vi "Predict(Dataset).vi"(6 "Dataset":T29={"Dataset_Size"=0, "Dims_In"={"C"=0, "H"=0, "W"=0}, "Labels"=[], "File Paths"=[], "Outputs Ref."=refnum, "Inputs Ref."=variant(refnum<data-value> refnum), "Dims_Out"={"C"=0, "H"=0, "W"=0}}, 8 "error in (no error)":errorcluster, 10 "Feature Scorer Params":T27, 11 "PCore_Instance in":T1={"Dataset_Stats"={"means"={"R"=0.0, "G"=0.0, "B"=0.0}, "vars"={"R"=0.0, "G"=0.0, "B"=0.0}, "DS_Size"=0}, "NN"={"Name"="", "No of Layers"=0, "mBatch"=0, "Layers"=[], "Dimty"=enum."In1D_Out1D", "Dims_In"={"C"=0, "H"=0, "W"=0}, "Dims_Out"={"C"=0, "H"=0, "W"=0}, "Working_Dir"=path "", "Train?"=FALSE, "Train_Params"={"Optimizer"=enum."SGD", "Beta_1"=0.0, "Beta_2"=0.0, "Weight Decay(L1)"=0.0, "Weight Decay(L2)"=0.0, "Data_Sampling"=enum."Random"}, "LR_Update_Policy"={"Policy_Type"=enum."Manual", "LR0"=0.0, "k"=0.0, "WarmUp_Policy"=enum."Step", "WarmUp_Iter"=0, "WarmUp_Ratio"=0.0}, "Session Data"={"Epochs"=0.0, "Tot_Iter"=0, "LR"=0.0, "LR_iter"=0}, "Ground_truth"={"Y"=variant}, "NNg_hdls"={"cudnn"=0, "cublas"=0, "stream"=0, "curand"=0}, "NN_Device"=enum."CPU", "GPU Id"=0, "Labels"=[], "Receptive Field"=[], "Loss_Type"=enum."None", "Loss_Cfg_Prms"=variant, "NNG_WS"={"NNG_WS_Mem"=refnum, "Max_WS_Size"=0}}, "PCore_Device"=enum."CPU", "PatchCore_Init_CFG"={"BackBone"=enum."WRN_50_2_L2L3", "Out_Layers_Names"=[], "Patch_Size"=0}, "Coreset Params"={"Sampling_Ratio"=0.0, "Startd_idx"=0, "Random_Proj?"=FALSE, "Rnd. Proj. Params"={"Proj._Dim."=0, "Epsilon"=0.9, "Seed"=42}}, "MemBank_Data"={"MemBank"=variant, "MemBank Norm"=variant}} {"NN out"."LR_Update_Policy"."WarmUp_Ratio" min=1; "NN out"."LR_Update_Policy"."WarmUp_Iter" min=1; "NN out"."LR_Update_Policy"."LR0" format="%.7f"; "Dataset_Stats"."vars"."R" format="%#_3g"; "Dataset_Stats"."vars"."G" format="%#_3g"; "Dataset_Stats"."vars"."B" format="%#_3g"; "Dataset_Stats"."means"."R" format="%#_3g"; "Dataset_Stats"."means"."G" format="%#_3g"; "Dataset_Stats"."means"."B" format="%#_3g"}) -> (0 "error out":errorcluster, 1 "anomaly maps":sgl[][][](array[numeric]), 2 "pred scores":sgl[](array[numeric]), 3 "PCore_Instance out":T1={"Dataset_Stats"={"means"={"R"=0.66, "G"=0.59, "B"=0.44}, "vars"={"R"=0.66, "G"=0.59, "B"=0.44}, "DS_Size"=0}, "NN"={"Name"="wrn", "No of Layers"=63, "mBatch"=1, "Layers"=[refnum, refnum, refnum, refnum, refnum, refnum, refnum, refnum, refnum, refnum, refnum, refnum, refnum, refnum, refnum, refnum, refnum, refnum, refnum, refnum, refnum, refnum, refnum, refnum, refnum, refnum, refnum, refnum, refnum, refnum, refnum, refnum, refnum, refnum, refnum, refnum, refnum, refnum, refnum, refnum, refnum, refnum, refnum, refnum, refnum, refnum, refnum, refnum, refnum, refnum, refnum, refnum, refnum, refnum, refnum, refnum, refnum, refnum, refnum, refnum, refnum, refnum, refnum], "Dimty"=enum."In3D_Out3D", "Dims_In"={"C"=3, "H"=224, "W"=224}, "Dims_Out"={"C"=302, "H"=28, "W"=28}, "Working_Dir"=path "D:/Ngene/Projects_SVN/DeepLTK/R_and_D/2024_02_01_Patchcore/LabVIEW/PatchCore_v5.0/working/wrn", "Train?"=FALSE, "Train_Params"={"Optimizer"=enum."SGD", "Beta_1"=0.999, "Beta_2"=0.999, "Weight Decay(L1)"=0.0, "Weight Decay(L2)"=0.0, "Data_Sampling"=enum."Random"}, "LR_Update_Policy"={"Policy_Type"=enum."Manual", "LR0"=0.0, "k"=0.0, "WarmUp_Policy"=enum."Step", "WarmUp_Iter"=100, "WarmUp_Ratio"=10.0}, "Session Data"={"Epochs"=0.0, "Tot_Iter"=1, "LR"=0.0, "LR_iter"=1}, "Ground_truth"={"Y"=variant(refnum<data-value> refnum)}, "NNg_hdls"={"cudnn"=2143106709504, "cublas"=2177817002560, "stream"=2141212075440, "curand"=2143055681792}, "NN_Device"=enum."GPU", "GPU Id"=0, "Labels"=["tench", "goldfish", "great white shark", "tiger shark", "hammerhead", "electric ray", "stingray", "cock", "hen", "ostrich", "brambling", "goldfinch", "house finch", "junco", "indigo bunting", "robin", "bulbul", "jay", "magpie", "chickadee", "water ouzel", "kite", "bald eagle", "vulture", "great grey owl", "European fire salamander", "common newt", "eft", "spotted salamander", "axolotl", "bullfrog", "tree frog", "tailed frog", "loggerhead", "leatherback turtle", "mud turtle", "terrapin", "box turtle", "banded gecko", "common iguana", "American chameleon", "whiptail", "agama", "frilled lizard", "alligator lizard", "Gila monster", "green lizard", "African chameleon", "Komodo dragon", "African crocodile", "American alligator", "triceratops", "thunder snake", "ringneck snake", "hognose snake", "green snake", "king snake", "garter snake", "water snake", "vine snake", "night snake", "boa constrictor", "rock python", "Indian cobra", "green mamba", "sea snake", "horned viper", "diamondback", "sidewinder", "trilobite", "harvestman", "scorpion", "black and gold garden spider", "barn spider", "garden spider", "black widow", "tarantula", "wolf spider", "tick", "centipede", "black grouse", "ptarmigan", "ruffed grouse", "prairie chicken", "peacock", "quail", "partridge", "African grey", "macaw", "sulphur-crested cockatoo", "lorikeet", "coucal", "bee eater", "hornbill", "hummingbird", "jacamar", "toucan", "drake", "red-breasted merganser", "goose", "black swan", "tusker", "echidna", "platypus", "wallaby", "koala", "wombat", "jellyfish", "sea anemone", "brain coral", "flatworm", "nematode", "conch", "snail", "slug", "sea slug", "chiton", "chambered nautilus", "Dungeness crab", "rock crab", "fiddler crab", "king crab", "American lobster", "spiny lobster", "crayfish", "hermit crab", "isopod", "white stork", "black stork", "spoonbill", "flamingo", "little blue heron", "American egret", "bittern", "crane", "limpkin", "European gallinule", "American coot", "bustard", "ruddy turnstone", "red-backed sandpiper", "redshank", "dowitcher", "oystercatcher", "pelican", "king penguin", "albatross", "grey whale", "killer whale", "dugong", "sea lion", "Chihuahua", "Japanese spaniel", "Maltese dog", "Pekinese", "Shih-Tzu", "Blenheim spaniel", "papillon", "toy terrier", "Rhodesian ridgeback", "Afghan hound", "basset", "beagle", "bloodhound", "bluetick", "black-and-tan coonhound", "Walker hound", "English foxhound", "redbone", "borzoi", "Irish wolfhound", "Italian greyhound", "whippet", "Ibizan hound", "Norwegian elkhound", "otterhound", "Saluki", "Scottish deerhound", "Weimaraner", "Staffordshire bullterrier", "American Staffordshire terrier", "Bedlington terrier", "Border terrier", "Kerry blue terrier", "Irish terrier", "Norfolk terrier", "Norwich terrier", "Yorkshire terrier", "wire-haired fox terrier", "Lakeland terrier", "Sealyham terrier", "Airedale", "cairn", "Australian terrier", "Dandie Dinmont", "Boston bull", "miniature schnauzer", "giant schnauzer", "standard schnauzer", "Scotch terrier", "Tibetan terrier", "silky terrier", "soft-coated wheaten terrier", "West Highland white terrier", "Lhasa", "flat-coated retriever", "curly-coated retriever", "golden retriever", "Labrador retriever", "Chesapeake Bay retriever", "German short-haired pointer", "vizsla", "English setter", "Irish setter", "Gordon setter", "Brittany spaniel", "clumber", "English springer", "Welsh springer spaniel", "cocker spaniel", "Sussex spaniel", "Irish water spaniel", "kuvasz", "schipperke", "groenendael", "malinois", "briard", "kelpie", "komondor", "Old English sheepdog", "Shetland sheepdog", "collie", "Border collie", "Bouvier des Flandres", "Rottweiler", "German shepherd", "Doberman", "miniature pinscher", "Greater Swiss Mountain dog", "Bernese mountain dog", "Appenzeller", "EntleBucher", "boxer", "bull mastiff", "Tibetan mastiff", "French bulldog", "Great Dane", "Saint Bernard", "Eskimo dog", "malamute", "Siberian husky", "dalmatian", "affenpinscher", "basenji", "pug", "Leonberg", "Newfoundland", "Great Pyrenees", "Samoyed", "Pomeranian", "chow", "keeshond", "Brabancon griffon", "Pembroke", "Cardigan", "toy poodle", "miniature poodle", "standard poodle", "Mexican hairless", "timber wolf", "white wolf", "red wolf", "coyote", "dingo", "dhole", "African hunting dog", "hyena", "red fox", "kit fox", "Arctic fox", "grey fox", "tabby", "tiger cat", "Persian cat", "Siamese cat", "Egyptian cat", "cougar", "lynx", "leopard", "snow leopard", "jaguar", "lion", "tiger", "cheetah", "brown bear", "American black bear", "ice bear", "sloth bear", "mongoose", "meerkat", "tiger beetle", "ladybug", "ground beetle", "long-horned beetle", "leaf beetle", "dung beetle", "rhinoceros beetle", "weevil", "fly", "bee", "ant", "grasshopper", "cricket", "walking stick", "cockroach", "mantis", "cicada", "leafhopper", "lacewing", "dragonfly", "damselfly", "admiral", "ringlet", "monarch", "cabbage butterfly", "sulphur butterfly", "lycaenid", "starfish", "sea urchin", "sea cucumber", "wood rabbit", "hare", "Angora", "hamster", "porcupine", "fox squirrel", "marmot", "beaver", "guinea pig", "sorrel", "zebra", "hog", "wild boar", "warthog", "hippopotamus", "ox", "water buffalo", "bison", "ram", "bighorn", "ibex", "hartebeest", "impala", "gazelle", "Arabian camel", "llama", "weasel", "mink", "polecat", "black-footed ferret", "otter", "skunk", "badger", "armadillo", "three-toed sloth", "orangutan", "gorilla", "chimpanzee", "gibbon", "siamang", "guenon", "patas", "baboon", "macaque", "langur", "colobus", "proboscis monkey", "marmoset", "capuchin", "howler monkey", "titi", "spider monkey", "squirrel monkey", "Madagascar cat", "indri", "Indian elephant", "African elephant", "lesser panda", "giant panda", "barracouta", "eel", "coho", "rock beauty", "anemone fish", "sturgeon", "gar", "lionfish", "puffer", "abacus", "abaya", "academic gown", "accordion", "acoustic guitar", "aircraft carrier", "airliner", "airship", "altar", "ambulance", "amphibian", "analog clock", "apiary", "apron", "ashcan", "assault rifle", "backpack", "bakery", "balance beam", "balloon", "ballpoint", "Band Aid", "banjo", "bannister", "barbell", "barber chair", "barbershop", "barn", "barometer", "barrel", "barrow", "baseball", "basketball", "bassinet", "bassoon", "bathing cap", "bath towel", "bathtub", "beach wagon", "beacon", "beaker", "bearskin", "beer bottle", "beer glass", "bell cote", "bib", "bicycle-built-for-two", "bikini", "binder", "binoculars", "birdhouse", "boathouse", "bobsled", "bolo tie", "bonnet", "bookcase", "bookshop", "bottlecap", "bow", "bow tie", "brass", "brassiere", "breakwater", "breastplate", "broom", "bucket", "buckle", "bulletproof vest", "bullet train", "butcher shop", "cab", "caldron", "candle", "cannon", "canoe", "can opener", "cardigan", "car mirror", "carousel", "carpenter's kit", "carton", "car wheel", "cash machine", "cassette", "cassette player", "castle", "catamaran", "CD player", "cello", "cellular telephone", "chain", "chainlink fence", "chain mail", "chain saw", "chest", "chiffonier", "chime", "china cabinet", "Christmas stocking", "church", "cinema", "cleaver", "cliff dwelling", "cloak", "clog", "cocktail shaker", "coffee mug", "coffeepot", "coil", "combination lock", "computer keyboard", "confectionery", "container ship", "convertible", "corkscrew", "cornet", "cowboy boot", "cowboy hat", "cradle", "crane", "crash helmet", "crate", "crib", "Crock Pot", "croquet ball", "crutch", "cuirass", "dam", "desk", "desktop computer", "dial telephone", "diaper", "digital clock", "digital watch", "dining table", "dishrag", "dishwasher", "disk brake", "dock", "dogsled", "dome", "doormat", "drilling platform", "drum", "drumstick", "dumbbell", "Dutch oven", "electric fan", "electric guitar", "electric locomotive", "entertainment center", "envelope", "espresso maker", "face powder", "feather boa", "file", "fireboat", "fire engine", "fire screen", "flagpole", "flute", "folding chair", "football helmet", "forklift", "fountain", "fountain pen", "four-poster", "freight car", "French horn", "frying pan", "fur coat", "garbage truck", "gasmask", "gas pump", "goblet", "go-kart", "golf ball", "golfcart", "gondola", "gong", "gown", "grand piano", "greenhouse", "grille", "grocery store", "guillotine", "hair slide", "hair spray", "half track", "hammer", "hamper", "hand blower", "hand-held computer", "handkerchief", "hard disc", "harmonica", "harp", "harvester", "hatchet", "holster", "home theater", "honeycomb", "hook", "hoopskirt", "horizontal bar", "horse cart", "hourglass", "iPod", "iron", "jack-o'-lantern", "jean", "jeep", "jersey", "jigsaw puzzle", "jinrikisha", "joystick", "kimono", "knee pad", "knot", "lab coat", "ladle", "lampshade", "laptop", "lawn mower", "lens cap", "letter opener", "library", "lifeboat", "lighter", "limousine", "liner", "lipstick", "Loafer", "lotion", "loudspeaker", "loupe", "lumbermill", "magnetic compass", "mailbag", "mailbox", "maillot", "maillot", "manhole cover", "maraca", "marimba", "mask", "matchstick", "maypole", "maze", "measuring cup", "medicine chest", "megalith", "microphone", "microwave", "military uniform", "milk can", "minibus", "miniskirt", "minivan", "missile", "mitten", "mixing bowl", "mobile home", "Model T", "modem", "monastery", "monitor", "moped", "mortar", "mortarboard", "mosque", "mosquito net", "motor scooter", "mountain bike", "mountain tent", "mouse", "mousetrap", "moving van", "muzzle", "nail", "neck brace", "necklace", "nipple", "notebook", "obelisk", "oboe", "ocarina", "odometer", "oil filter", "organ", "oscilloscope", "overskirt", "oxcart", "oxygen mask", "packet", "paddle", "paddlewheel", "padlock", "paintbrush", "pajama", "palace", "panpipe", "paper towel", "parachute", "parallel bars", "park bench", "parking meter", "passenger car", "patio", "pay-phone", "pedestal", "pencil box", "pencil sharpener", "perfume", "Petri dish", "photocopier", "pick", "pickelhaube", "picket fence", "pickup", "pier", "piggy bank", "pill bottle", "pillow", "ping-pong ball", "pinwheel", "pirate", "pitcher", "plane", "planetarium", "plastic bag", "plate rack", "plow", "plunger", "Polaroid camera", "pole", "police van", "poncho", "pool table", "pop bottle", "pot", "potter's wheel", "power drill", "prayer rug", "printer", "prison", "projectile", "projector", "puck", "punching bag", "purse", "quill", "quilt", "racer", "racket", "radiator", "radio", "radio telescope", "rain barrel", "recreational vehicle", "reel", "reflex camera", "refrigerator", "remote control", "restaurant", "revolver", "rifle", "rocking chair", "rotisserie", "rubber eraser", "rugby ball", "rule", "running shoe", "safe", "safety pin", "saltshaker", "sandal", "sarong", "sax", "scabbard", "scale", "school bus", "schooner", "scoreboard", "screen", "screw", "screwdriver", "seat belt", "sewing machine", "shield", "shoe shop", "shoji", "shopping basket", "shopping cart", "shovel", "shower cap", "shower curtain", "ski", "ski mask", "sleeping bag", "slide rule", "sliding door", "slot", "snorkel", "snowmobile", "snowplow", "soap dispenser", "soccer ball", "sock", "solar dish", "sombrero", "soup bowl", "space bar", "space heater", "space shuttle", "spatula", "speedboat", "spider web", "spindle", "sports car", "spotlight", "stage", "steam locomotive", "steel arch bridge", "steel drum", "stethoscope", "stole", "stone wall", "stopwatch", "stove", "strainer", "streetcar", "stretcher", "studio couch", "stupa", "submarine", "suit", "sundial", "sunglass", "sunglasses", "sunscreen", "suspension bridge", "swab", "sweatshirt", "swimming trunks", "swing", "switch", "syringe", "table lamp", "tank", "tape player", "teapot", "teddy", "television", "tennis ball", "thatch", "theater curtain", "thimble", "thresher", "throne", "tile roof", "toaster", "tobacco shop", "toilet seat", "torch", "totem pole", "tow truck", "toyshop", "tractor", "trailer truck", "tray", "trench coat", "tricycle", "trimaran", "tripod", "triumphal arch", "trolleybus", "trombone", "tub", "turnstile", "typewriter keyboard", "umbrella", "unicycle", "upright", "vacuum", "vase", "vault", "velvet", "vending machine", "vestment", "viaduct", "violin", "volleyball", "waffle iron", "wall clock", "wallet", "wardrobe", "warplane", "washbasin", "washer", "water bottle", "water jug", "water tower", "whiskey jug", "whistle", "wig", "window screen", "window shade", "Windsor tie", "wine bottle", "wing", "wok", "wooden spoon", "wool", "worm fence", "wreck", "yawl", "yurt", "web site", "comic book", "crossword puzzle", "street sign", "traffic light", "book jacket", "menu", "plate", "guacamole", "consomme", "hot pot", "trifle", "ice cream", "ice lolly", "French loaf", "bagel", "pretzel", "cheeseburger", "hotdog", "mashed potato", "head cabbage", "broccoli", "cauliflower", "zucchini", "spaghetti squash", "acorn squash", "butternut squash", "cucumber", "artichoke", "bell pepper", "cardoon", "mushroom", "Granny Smith", "strawberry", "orange", "lemon", "fig", "pineapple", "banana", "jackfruit", "custard apple", "pomegranate", "hay", "carbonara", "chocolate sauce", "dough", "meat loaf", "pizza", "potpie", "burrito", "red wine", "espresso", "cup", "eggnog", "alp", "bubble", "cliff", "coral reef", "geyser", "lakeside", "promontory", "sandbar", "seashore", "valley", "volcano", "ballplayer", "groom", "scuba diver", "rapeseed", "daisy", "yellow lady's slipper", "corn", "acorn", "hip", "buckeye", "coral fungus", "agaric", "gyromitra", "stinkhorn", "earthstar", "hen-of-the-woods", "bolete", "ear", "toilet tissue"], "Receptive Field"=[{"V"=1, "H"=1}, {"V"=7, "H"=7}, {"V"=9, "H"=9}, {"V"=9, "H"=9}, {"V"=21, "H"=21}, {"V"=21, "H"=21}, {"V"=9, "H"=9}, {"V"=21, "H"=21}, {"V"=21, "H"=21}, {"V"=33, "H"=33}, {"V"=33, "H"=33}, {"V"=33, "H"=33}, {"V"=33, "H"=33}, {"V"=45, "H"=45}, {"V"=45, "H"=45}, {"V"=45, "H"=45}, {"V"=45, "H"=45}, {"V"=57, "H"=57}, {"V"=57, "H"=57}, {"V"=45, "H"=45}, {"V"=57, "H"=57}, {"V"=57, "H"=57}, {"V"=81, "H"=81}, {"V"=81, "H"=81}, {"V"=81, "H"=81}, {"V"=81, "H"=81}, {"V"=105, "H"=105}, {"V"=105, "H"=105}, {"V"=105, "H"=105}, {"V"=105, "H"=105}, {"V"=129, "H"=129}, {"V"=129, "H"=129}, {"V"=129, "H"=129}, {"V"=129, "H"=129}, {"V"=153, "H"=153}, {"V"=153, "H"=153}, {"V"=129, "H"=129}, {"V"=153, "H"=153}, {"V"=153, "H"=153}, {"V"=201, "H"=201}, {"V"=201, "H"=201}, {"V"=201, "H"=201}, {"V"=201, "H"=201}, {"V"=249, "H"=249}, {"V"=249, "H"=249}, {"V"=249, "H"=249}, {"V"=249, "H"=249}, {"V"=297, "H"=297}, {"V"=297, "H"=297}, {"V"=297, "H"=297}, {"V"=297, "H"=297}, {"V"=345, "H"=345}, {"V"=345, "H"=345}, {"V"=345, "H"=345}, {"V"=345, "H"=345}, {"V"=393, "H"=393}, {"V"=393, "H"=393}, {"V"=393, "H"=393}, {"V"=153, "H"=153}, {"V"=441, "H"=441}, {"V"=441, "H"=441}, {"V"=441, "H"=441}, {"V"=441, "H"=441}], "Loss_Type"=enum."MSE", "Loss_Cfg_Prms"=variant, "NNG_WS"={"NNG_WS_Mem"=refnum, "Max_WS_Size"=-1}}, "PCore_Device"=enum."GPU(CuLab)", "PatchCore_Init_CFG"={"BackBone"=enum."WRN_50_2_L2L3", "Out_Layers_Names"=[], "Patch_Size"=0}, "Coreset Params"={"Sampling_Ratio"=0.0, "Startd_idx"=0, "Random_Proj?"=FALSE, "Rnd. Proj. Params"={"Proj._Dim."=0, "Epsilon"=0.9, "Seed"=42}}, "MemBank_Data"={"MemBank"=variant, "MemBank Norm"=variant}} {"NN out"."LR_Update_Policy"."WarmUp_Ratio" min=1; "NN out"."LR_Update_Policy"."WarmUp_Iter" min=1; "NN out"."LR_Update_Policy"."LR0" format="%.7f"; "Dataset_Stats"."vars"."R" format="%#_3g"; "Dataset_Stats"."vars"."G" format="%#_3g"; "Dataset_Stats"."vars"."B" format="%#_3g"; "Dataset_Stats"."means"."R" format="%#_3g"; "Dataset_Stats"."means"."G" format="%#_3g"; "Dataset_Stats"."means"."B" format="%#_3g"}, 5 "dT_Predict(Dataset)":dbl)   [LabVIEW 2020]
doc: "Runs forward propagation over whole dataset of type In3D_Out3D and returns prediction for a pretrained network.\n\n<b>NN in</b> - Network instance input.\n<b>Dataset</b> - A dataset of type In3D_Out3D for which predictions should be generated.\n<b>Predictions</b> - Contains feature maps of the last layer (predictions).\n<b>Predictions</b> - Returns predictions (network outputs) for applied dataset.\n<b>NN out</b> - Network instance output."
uses:
  <vilib>/Ngene/Deep Learning Toolkit/Toolkit/NN_Data/API/DataSet/DataSet_Types/NN_DataSet(In3D_Out3D).ctl
  <vilib>/Ngene/Deep Learning Toolkit/Toolkit/NN_Data/API/NN_Dims(C,H,W).ctl
  <vilib>/Ngene/Deep Learning Toolkit/Toolkit/NN_Data/Controls/DataRef_Types/4D/NN_Data_ref(4D_SGL).ctl
  API/Controls/PatchCore_Instance.ctl
  API/Controls/PatchCore_DS_Stats.ctl
  API/Controls/Image_Stats_RGB.ctl
  <vilib>/Ngene/Deep Learning Toolkit/Toolkit/NN_Network/Controls/NN.ctl
  <vilib>/Ngene/Deep Learning Toolkit/Toolkit/NN_Layers/Controls/NN_Layer_ref.ctl
  <vilib>/Ngene/Deep Learning Toolkit/Toolkit/NN_Layers/Controls/NN_Layer.ctl
  <vilib>/Ngene/Deep Learning Toolkit/Toolkit/NN_Layers/Controls/NN_Layer_Type.ctl
  <vilib>/Ngene/Deep Learning Toolkit/Toolkit/NN_Layers/Controls/NN_Layer_Metrics.ctl
  <vilib>/Ngene/Deep Learning Toolkit/Toolkit/NN_Network/Controls/NN_Device.ctl
  <vilib>/Ngene/Deep Learning Toolkit/Toolkit/NNg/cuda/Controls/nng_cuda_handles.ctl
  <vilib>/Ngene/Deep Learning Toolkit/Toolkit/NN_Layers/Controls/NN_Layer_Dimty.ctl
  <vilib>/Ngene/Deep Learning Toolkit/Toolkit/NN_Layers/Controls/NN_Layer_RF_State.ctl
  <vilib>/Ngene/Deep Learning Toolkit/Toolkit/NN_Data/API/NN_Dims(V,H).ctl
  <vilib>/Ngene/Deep Learning Toolkit/Toolkit/NN_Network/Controls/NN_In_Out_Dim-ty.ctl
  <vilib>/Ngene/Deep Learning Toolkit/Toolkit/NN_Train/Controls/NN_Train_Params.ctl
  <vilib>/Ngene/Deep Learning Toolkit/Toolkit/NN_Train/Controls/NN_Train_Optimizer.ctl
  <vilib>/Ngene/Deep Learning Toolkit/Toolkit/NN_Train/Controls/NN_Train_Data_Sampling.ctl
  <vilib>/Ngene/Deep Learning Toolkit/Toolkit/NN_Train/Controls/NN_LR_Policy_Cfg.ctl
  <vilib>/Ngene/Deep Learning Toolkit/Toolkit/NN_Train/Controls/NN_LR_Policy_Type.ctl
  <vilib>/Ngene/Deep Learning Toolkit/Toolkit/NN_Train/Controls/NN_Train_Session_Data.ctl
  <vilib>/Ngene/Deep Learning Toolkit/Toolkit/NN_Data/Controls/NN_Ground_truth.ctl
  <vilib>/Ngene/Deep Learning Toolkit/Toolkit/NN_Train/Controls/NN_Loss_Type.ctl
  <vilib>/Ngene/Deep Learning Toolkit/Toolkit/NNg/Network/WS/Controls/NNG_WS.ctl
  <vilib>/Ngene/Deep Learning Toolkit/Toolkit/NNg/Network/WS/Controls/NNg_WS_Mem_DVR.ctl
  <vilib>/Ngene/Deep Learning Toolkit/Toolkit/NNg/cuda/Controls/cuda_Mem_desc.ctl
  API/Controls/PCore_Device.ctl
  API/Controls/PatchCore_Init_CFG.ctl
  API/Controls/PatchCore_BackBone_Selector.ctl
  API/Controls/Coreset_Params.ctl
  API/Controls/Random_Projection_Coreset.ctl
  API/Controls/MemBank_and_Norm_Variants.ctl
  API/Controls/Feature_Scorer_Params.ctl
  API/Controls/Gaussian_Blur.ctl
  <vilib>/Ngene/Deep Learning Toolkit/Toolkit/NN_Data/subVIs/Get_Data_Vals/4D/NN_Data_Get_ValByRef(4D_SGL).vi
  <vilib>/Ngene/Deep Learning Toolkit/Toolkit/Deep_Learning_Toolkit_by_Ngene.lvlib
panel:
  out "anomaly map test":sgl[][][](array[numeric])
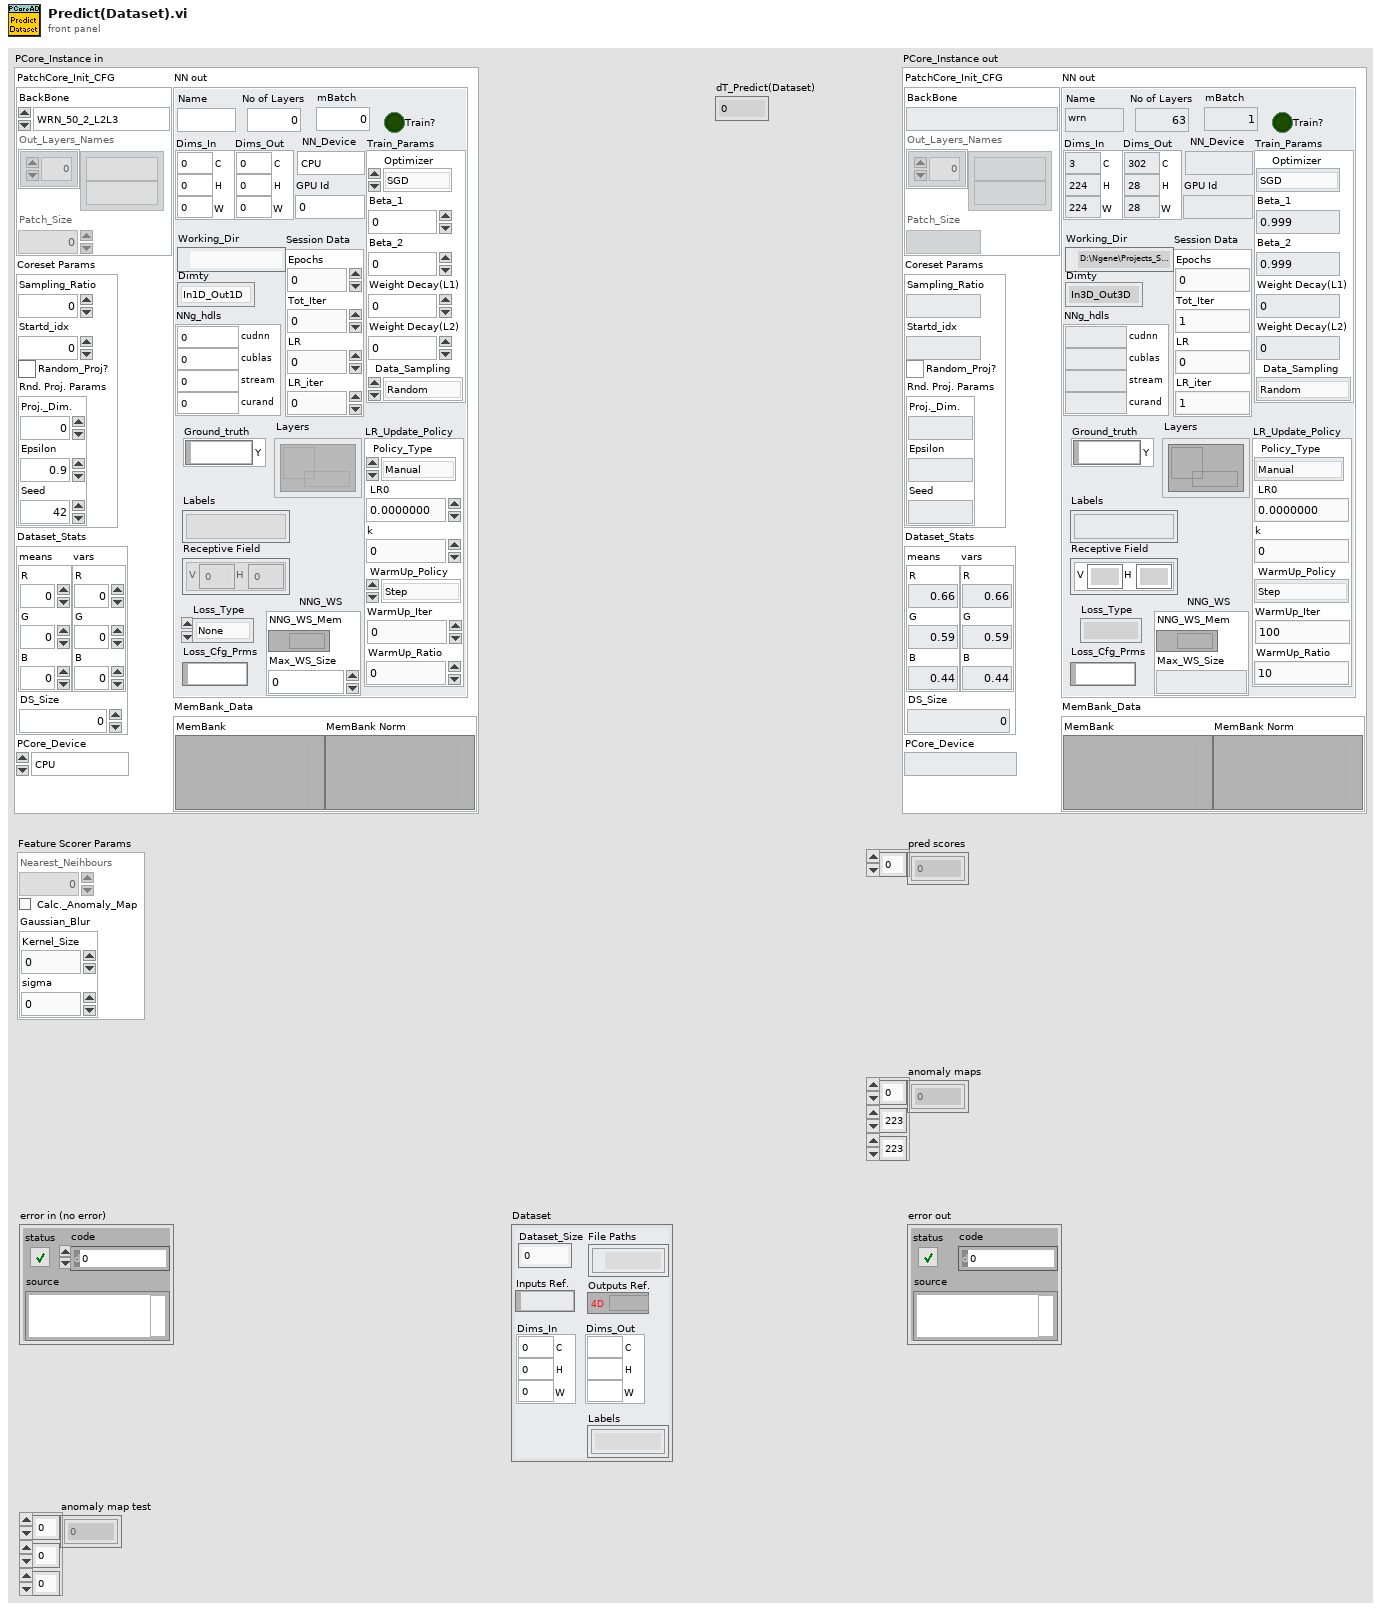
[diagram p1: front panel]
types:
  T1 = typedef "PatchCore_Instance.ctl" = cluster{"Dataset_Stats":T2, "NN":T4, "PCore_Device":T21, "PatchCore_Init_CFG":T22, "Coreset Params":T24, "MemBank_Data":T26}
  T2 = typedef "PatchCore_DS_Stats.ctl" = cluster{"means":T3, "vars":T3, "DS_Size":i32}
  T3 = typedef "Image_Stats_RGB.ctl" = cluster{"R":sgl, "G":sgl, "B":sgl}
  T4 = typedef "Deep_Learning_Toolkit_by_Ngene.lvlib/NN.ctl" = cluster{"Name":string, "No of Layers":i32, "mBatch":i32, "Layers":T5[], "Dimty":T6, "Dims_In":T7, "Dims_Out":T7, "Working_Dir":path, "Train?":bool, "Train_Params":T8, "LR_Update_Policy":T11, "Session Data":T13, "Ground_truth":T14, "NNg_hdls":T15, "NN_Device":T16, "GPU Id":i32, "Labels":string[], "Receptive Field":T17[], "Loss_Type":T18, "Loss_Cfg_Prms":variant, "NNG_WS":T19}
  T5 = typedef "Deep_Learning_Toolkit_by_Ngene.lvlib/NN_Layer_ref.ctl" = refnum<data-value>
  T6 = typedef "Deep_Learning_Toolkit_by_Ngene.lvlib/NN_In_Out_Dim-ty.ctl" = enum8{"In1D_Out1D", "In3D_Out1D", "In3D_Out3D", "In3D_OutBBox"}
  T7 = typedef "Deep_Learning_Toolkit_by_Ngene.lvlib/NN_Dims(C,H,W).ctl" = cluster{"C":i32, "H":i32, "W":i32}
  T8 = typedef "Deep_Learning_Toolkit_by_Ngene.lvlib/NN_Train_Params.ctl" = cluster{"Optimizer":T9, "Beta_1":sgl, "Beta_2":sgl, "Weight Decay(L1)":sgl, "Weight Decay(L2)":sgl, "Data_Sampling":T10}
  T9 = typedef "Deep_Learning_Toolkit_by_Ngene.lvlib/NN_Train_Optimizer.ctl" = enum16{"SGD", "Adam", "Adagrad", "Adadelta", "RMSProp", "Nesterov"}
  T10 = typedef "Deep_Learning_Toolkit_by_Ngene.lvlib/NN_Train_Data_Sampling.ctl" = enum16{"Random", "Sequential"}
  T11 = typedef "Deep_Learning_Toolkit_by_Ngene.lvlib/NN_LR_Policy_Cfg.ctl" = cluster{"Policy_Type":T12, "LR0":dbl, "k":sgl, "WarmUp_Policy":enum16{"Step", "Ramp"}, "WarmUp_Iter":i32, "WarmUp_Ratio":sgl}
  T12 = typedef "Deep_Learning_Toolkit_by_Ngene.lvlib/NN_LR_Policy_Type.ctl" = enum16{"Manual", "Step", "Exp", "1/t"}
  T13 = typedef "Deep_Learning_Toolkit_by_Ngene.lvlib/NN_Train_Session_Data.ctl" = cluster{"Epochs":sgl, "Tot_Iter":i32, "LR":sgl, "LR_iter":i32}
  T14 = typedef "Deep_Learning_Toolkit_by_Ngene.lvlib/NN_Ground_truth.ctl" = cluster{"Y":variant}
  T15 = typedef "Deep_Learning_Toolkit_by_Ngene.lvlib/nng_cuda_handles.ctl" = cluster{"cudnn":u64, "cublas":u64, "stream":u64, "curand":u64}
  T16 = typedef "Deep_Learning_Toolkit_by_Ngene.lvlib/NN_Device.ctl" = enum16{"CPU", "GPU"}
  T17 = typedef "Deep_Learning_Toolkit_by_Ngene.lvlib/NN_Dims(V,H).ctl" = cluster{"V":i32, "H":i32}
  T18 = typedef "Deep_Learning_Toolkit_by_Ngene.lvlib/NN_Loss_Type.ctl" = enum16{"None", "MSE", "CrossEntropy", "YOLO_v2", "YOLO_v4"}
  T19 = typedef "Deep_Learning_Toolkit_by_Ngene.lvlib/NNG_WS.ctl" = cluster{"NNG_WS_Mem":T20, "Max_WS_Size":i64}
  T20 = typedef "Deep_Learning_Toolkit_by_Ngene.lvlib/NNg_WS_Mem_DVR.ctl" = refnum<data-value>
  T21 = typedef "PCore_Device.ctl" = enum16{"CPU", "GPU(CuLab)"}
  T22 = typedef "PatchCore_Init_CFG.ctl" = cluster{"BackBone":T23, "Out_Layers_Names":string[], "Patch_Size":u32}
  T23 = typedef "PatchCore_BackBone_Selector.ctl" = enum16{"WRN_50_2_L2L3"}
  T24 = typedef "Coreset_Params.ctl" = cluster{"Sampling_Ratio":sgl, "Startd_idx":i32, "Random_Proj?":bool, "Rnd. Proj. Params":T25}
  T25 = typedef "Random_Projection_Coreset.ctl" = cluster{"Proj._Dim.":i32, "Epsilon":sgl, "Seed":i32}
  T26 = typedef "MemBank_and_Norm_Variants.ctl" = cluster{"MemBank":variant, "MemBank Norm":variant}
  T27 = typedef "Feature_Scorer_Params.ctl" = cluster{"Nearest_Neihbours":i32, "Calculate Anomaly Map":bool, "Gaussian_Blur":T28}
  T28 = typedef "Gaussian_Blur.ctl" = cluster{"Kernel_Size":i32, "sigma":sgl}
  T29 = typedef "Deep_Learning_Toolkit_by_Ngene.lvlib/NN_DataSet(In3D_Out3D).ctl" = cluster{"Dataset_Size":i32, "Dims_In":T7, "Labels":string[], "File Paths":path[], "Outputs Ref.":T30, "Inputs Ref.":variant, "Dims_Out":T7}
  T30 = typedef "Deep_Learning_Toolkit_by_Ngene.lvlib/NN_Data_ref(4D_SGL).ctl" = refnum<data-value>
  T31 = typedef "Deep_Learning_Toolkit_by_Ngene.lvlib/NN_Layer.ctl" = cluster{"Name":string, "Layer_Data":variant, "Layer_Type":T32, "Dims_In":T7, "Layers_In":variant, "Dims_Out":T7, "Layers_Out":variant, "Metrics":T33, "GPU_Data":variant, "mBatch":i32, "NN_Device":T16, "NNg_hdls":T15, "Train?":bool, "Dimty":T34, "RecptField":T35}
  T32 = typedef "Deep_Learning_Toolkit_by_Ngene.lvlib/NN_Layer_Type.ctl" = enum16{"Input1D", "Input3D", "Conv1D", "Conv2D", "Conv2D_Adv", "MaxPool", "AvgPool", "UpSample", "DropOut3D", "ShortCut", "Concat", "SoftMax3D", "FC", "DropOut", "Softmax", "Flatten", "YOLO_v2", "YOLO_v4", "Activation", "BatchNormalization", "Unsupported"}
  T33 = typedef "Deep_Learning_Toolkit_by_Ngene.lvlib/NN_Layer_Metrics.ctl" = cluster{"Data":dbl, "Params":dbl, "Ops":dbl}
  T34 = typedef "Deep_Learning_Toolkit_by_Ngene.lvlib/NN_Layer_Dimty.ctl" = enum16{"1D", "3D"}
  T35 = typedef "Deep_Learning_Toolkit_by_Ngene.lvlib/NN_Layer_RF_State.ctl" = cluster{"Dims":T17, "J":T17}
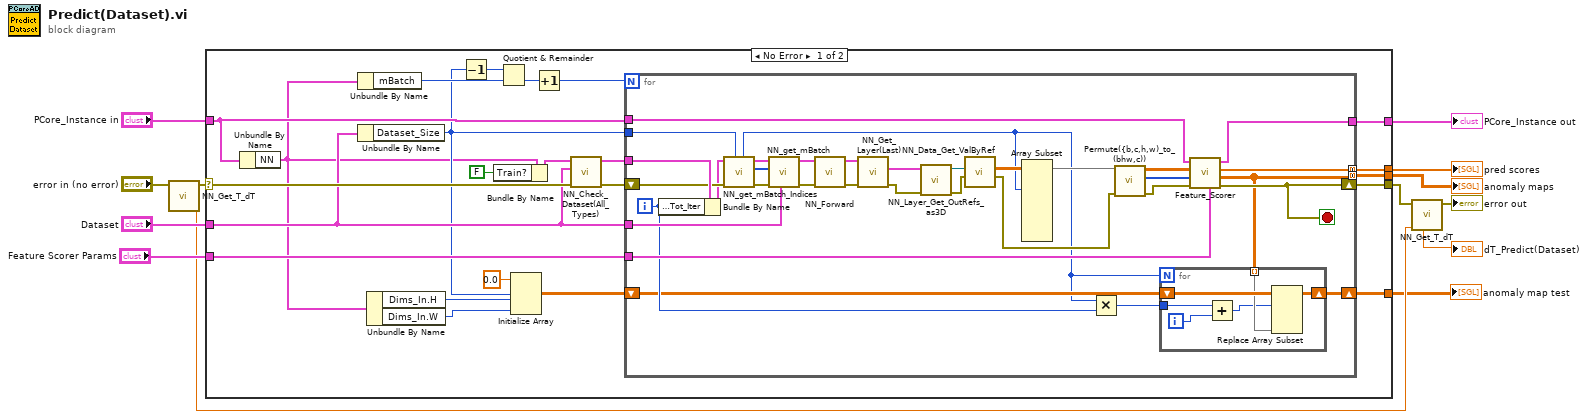
[diagram p0: block diagram]
diagram:
  n1 = call <vilib>:"NN_Get_T_dT.vi"("error in (no error)"="error in (no error)") -> ("T_out"=w4:dbl, "error out"=w6:errorcluster)  [unwired: 6 in, 1 out]
  n2 = case shown="No Error" w6 {
    selector: w6 -> [w28 w77]
    tunnel: "Dataset" -> [w26 _]
    tunnel: [w36 w77] -> w11
    tunnel: "PCore_Instance in" -> [w25 w76]
    tunnel: [w24 _] -> w9
    tunnel: [w23 _] -> w2
    tunnel: "Feature Scorer Params" -> [w22 _]
    tunnel: [w21 w76] -> w7
    tunnel: [w14 _] -> w1
    frame No Error {
      n3 = Unbundle By Name(w25) -> ("NN"=w18:T4)
      n4 = Unbundle By Name(w18) -> ("mBatch"=w30:i32)
      n5 = Unbundle By Name(w26) -> ("Dataset_Size"=w19:i32)
      n6 = Unbundle By Name(w18) -> ("Dims_In.H"=w17:i32, "Dims_In.W"=w16:i32)
      n7 = Decrement(x=w19) -> (x-1=w33:i32)
      n8 = Bundle By Name(cluster=w18, "Train?"=FALSE) -> (w35:T4)
      n9 = Quotient & Remainder(x=w33, y=w30) -> (floor(x/y)=w32:i32)  [unwired: 1 out]
      n10 = Initialize Array(sgl 0.0 ("element"), w19, w17, w16) -> (w15:sgl[][][])
      n11 = Increment(x=w32) -> (x+1=w31:i32)
      n12 = call <vilib>:"NN_Check_Dataset(All_Types).vi"("error in (no error)"=w28, "Train DataSet"=w26, "NN in"=w35) -> ("error out"=w27:errorcluster, "NN out"=w29:T4)  [unwired: 5 in, 2 out]
      n13 = for {
        N: w31 -> [_]
        shift-right: [w47] -> w36
        shift-left: w27 -> [w59]
        tunnel: w26 -> [w57]
        tunnel: w29 -> [w68]
        tunnel: w19 -> [w55]
        tunnel: w25 -> [w48]
        tunnel: [w46] -> w24 mode=concatenating
        tunnel: [w40] -> w23 mode=concatenating
        tunnel: w22 -> [w45]
        tunnel: [w44] -> w21
        shift-right: [w38] -> w14
        shift-left: w15 -> [w41]
        i -> [w42]
        stop <- w47 stop-if-true
        n14 = Bundle By Name(cluster=w68, "Session Data.Tot_Iter"=w42) -> (w56:T4)
        n15 = call <vilib>:"NN_get_mBatch_Indices.vi"("Dataset_Size"=w55, "error in (no error)"=w59, "NN in"=w56) -> ("error out"=w58:errorcluster, "Indices"=w54:i32[], "NN Out"=w60:T4, "Actual mBatch Size"=w37:i32)  [unwired: 5 in]
        n16 = call <vilib>:"NN_get_mBatch.vi"("DataSet"=w57, "error in (no error)"=w58, "Indices"=w54, "NN in"=w60) -> ("error out"=w66:errorcluster, "NN Out"=w67:T4)  [unwired: 5 in, 1 out]
        n17 = call <vilib>:"NN_Forward.vi"("error in (no error)"=w66, "NN in"=w67) -> ("error out"=w65:errorcluster, "NN out"=w69:T4)  [unwired: 6 in, 2 out]
        n18 = call <vilib>:"NN_Get_Layer(Last).vi"("error in (no error)"=w65, "NN in"=w69) -> ("error out"=w64:errorcluster, "Last_Layer"=w63:T31)  [unwired: 6 in, 2 out]
        n19 = call <vilib>:"NN_Layer_Get_OutRefs_as3D.vi"("error in (no error)"=w64, "Layer"=w63) -> ("error out"=w61:errorcluster, "Out"=w62:T30)  [unwired: 7 in, 1 out]
        n20 = call-poly <vilib>:"NN_Data_Get_ValByRef.vi"("error in (no error)"=w61, "DVR(4D_SGL)"=w62) -> ("error out"=w52:errorcluster, "Value(4D_SGL)"=w53:sgl[][][][])  [unwired: 6 in]
        n21 = Array Subset(array=w53, length (dim 0)=w37) -> (w43:sgl[][][][])  [unwired: 7 in]
        n22 = Multiply(x=w37, y=w42) -> (x*y=w39:i32)
        n23 = call "Permute({b,c,h,w)_to_(bhw,c)).vi"("error in"=w52, "Features (bs, (c1+c2+...+cN), h, w)"=w43) -> ("error out"=w50:errorcluster, "Orig dims (bs, h, w, (c1+c2+...+cN))"=w49:i32[], "Features resshaped ((bs  x h x w),  c1+c1+..+ cN, )"=w51:sgl[][])  [unwired: 6 in, 1 out]
        n24 = call "Feature_Scorer.vi"("Feature Scorer Params"=w45, "error in"=w50, "bs, h, w, c1+..cN"=w49, "embedding"=w51, "PCore_Instance in"=w48) -> ("error out"=w47:errorcluster, "anomaly map"=w40:sgl[][][], "pred score"=w46:sgl[], "PCore_Instance out"=w44:T1)  [unwired: 2 in, 1 out]
        n25 = for {
          N: w37 -> [_]
          tunnel: w40 -> [w74] mode=indexing
          tunnel: w39 -> [w73]
          shift-right: [w72] -> w38
          shift-left: w41 -> [w75]
          i -> [w71]
          n26 = Add(x=w73, y=w71) -> (x+y=w70:i32)
          n27 = Replace Array Subset(array=w75, new element=w74, index (dim 0)=w70) -> (w72:sgl[][][])  [unwired: 2 in]
        }
      }
    }
    frame Error {
    }
  }
  "pred scores" <- w9
  "anomaly maps" <- w2
  "PCore_Instance out" <- w7
  "anomaly map test" <- w1
  n28 = call <vilib>:"NN_Get_T_dT.vi"("T_in"=w4, "error in (no error)"=w11) -> ("error out"=→"error out":errorcluster, "dT"=→"dT_Predict(Dataset)":dbl)  [unwired: 5 in, 1 out]
